vi "Class.vi"(7 "Set? (f)":bool, 11 "DaqMx_Single in":refnum<class "DaqMx_Single.lvclass">) -> (3 "DaqMx_Single out":refnum<class "DaqMx_Single.lvclass">)   [LabVIEW 2018, in "FgenPlugins.lvlib" / "DaqMx_Single.lvclass"]
uses:
  DaqMx_Single.lvclass
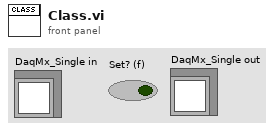
[diagram p1: front panel]
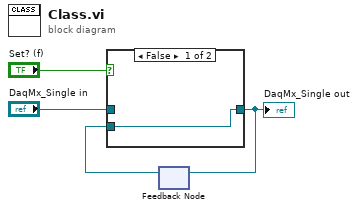
[diagram p0: block diagram]
diagram:
  n1 = feedback #1() -> (w1:refnum<class "DaqMx_Single.lvclass">)  [unwired: 1 in]
  n2 = case shown="False" "Set? (f)" {
    tunnel: "DaqMx_Single in" -> [_ w6]
    tunnel: [w5 w6] -> w3
    tunnel: w1 -> [w5 _]
    frame False {
    }
    frame True {
    }
  }
  "DaqMx_Single out" <- w3
  n3 = feedback-in #1(w3) -> ()
